vi "draw.vi"(0 "reference":refnum<class "PackageNode.lvclass">, 1 "graphics":refnum<class "Graphics.lvclass">, 5 "error in (no error)":errorcluster) -> (14 "reference out":refnum<class "PackageNode.lvclass">, 19 "error out":errorcluster)   [LabVIEW 2014, in "PackageNode.lvclass"]
doc: "public void draw(Graphics2D g2)"
uses:
  <resource>/Framework/Providers/Open_GDS/UML/PackageNode_class/PackageNode.lvclass
  <resource>/Framework/Providers/Open_GDS/UML/Graphics_class/Graphics.lvclass
  <resource>/Framework/Providers/Open_GDS/UML/General/Point/Point Point2D.ctl
  <resource>/Framework/Providers/Open_GDS/UML/MultiLineString_class/MultiLineString.lvclass
  <resource>/Framework/Providers/Open_GDS/UML/RectangularNode_class/RectangularNode.lvclass
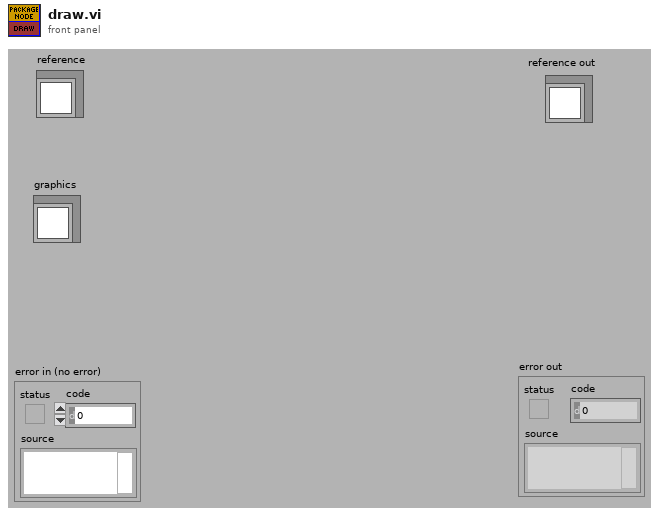
[diagram p1: front panel]
types:
  T1 = typedef "Point Point2D.ctl" = cluster{"x":dbl, "y":dbl}
  T2 = typedef "PackageNode.lvclass/ObjectAttributes.ctl" = cluster{"name":string, "contents":refnum<class "MultiLineString.lvclass">, "DEFAULT_TOP_WIDTH":i32, "DEFAULT_TOP_HEIGHT":i32, "DEFAULT_WIDTH":i32, "DEFAULT_HEIGHT":i32, "NAME_GAP":i32, "XGAP":i32, "YGAP":i32, "Collapsed":bool, "Note color":u32, "Justification":u16}
  T3 = typedef "RectangularNode.lvclass/ObjectAttributes.ctl" = cluster{"bounds":T4}
  T4 = typedef "Rectangle Rectangle2D.ctl" = cluster{"x":dbl, "y":dbl, "width":dbl, "height":dbl}
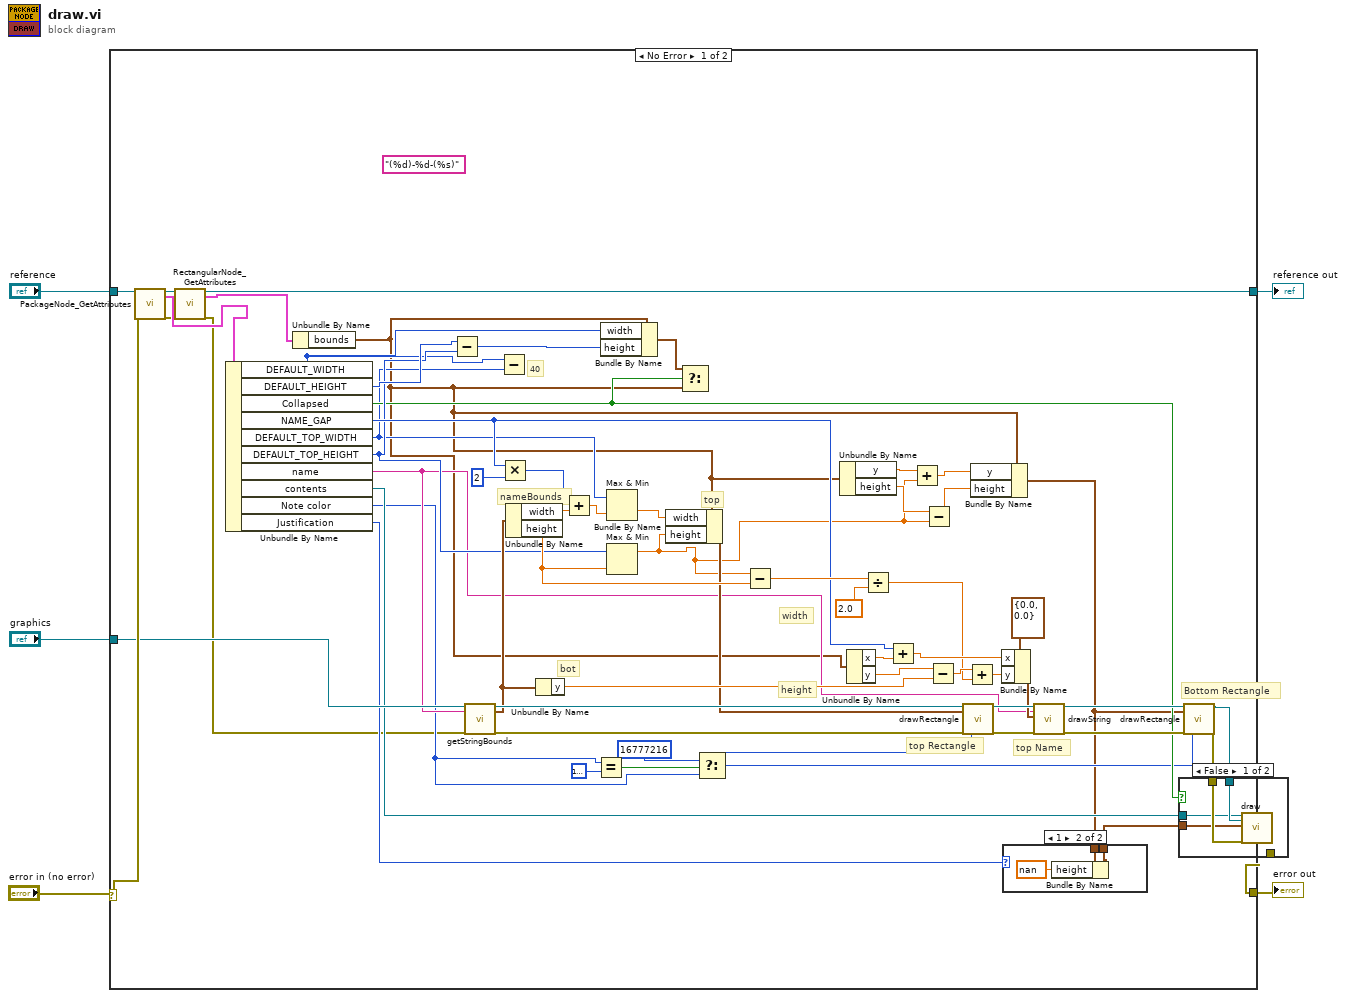
[diagram p0: block diagram]
diagram:
  n1 = case shown="No Error" "error in (no error)" {
    selector: "error in (no error)" -> [w64 w77]
    tunnel: "reference" -> [w66 w78]
    tunnel: [w65 w77] -> w4
    tunnel: [w7 w78] -> w3
    tunnel: "graphics" -> [w63 _]
    frame No Error {
      (unwired) "(%d)-%d-(%s)" ("format string")
      # "40"
      # "Bottom Rectangle"
      # "top Name"
      # "top Rectangle"
      # "height"
      # "width"
      # "bot"
      # "top"
      # "nameBounds"
      n2 = call <resource>:"PackageNode_GetAttributes.vi"("reference in"=w66, "error in (no error)"=w64) -> ("reference out"=w10:refnum<class "PackageNode.lvclass">, "Data"=w11:T2, "error out"=w9:errorcluster)  [unwired: 1 in, 14 out]
      n3 = call <resource>:"RectangularNode_GetAttributes.vi"("reference in"=w10, "error in (no error)"=w9) -> ("reference out"=w7:refnum<class "PackageNode.lvclass">, "Data"=w6:T3, "error out"=w8:errorcluster)  [unwired: 14 in, 1 out]
      n4 = Unbundle By Name(w11) -> ("DEFAULT_WIDTH"=w22:i32, "DEFAULT_HEIGHT"=w27:i32, "Collapsed"=w24:bool, "NAME_GAP"=w38:i32, "DEFAULT_TOP_WIDTH"=w21:i32, "DEFAULT_TOP_HEIGHT"=w26:i32, "name"=w23:string, "contents"=w29:refnum<class "MultiLineString.lvclass">, "Note color"=w16:u32, "Justification"=w12:u16)
      n5 = Unbundle By Name(w6) -> ("bounds"=w20:T4)
      n6 = Subtract(x=w27, y=w26) -> (x-y=w25:i32)
      n7 = call-dynamic "getStringBounds.vi"("reference"=w63, "text"=w23, "error in (no error)"=w8) -> ("reference out"=w60:refnum<class "Graphics.lvclass">, "bounds"=w36:T4, "error out"=w39:errorcluster)  [unwired: 14 in]
      n8 = Subtract(x=w22, y=w21) -> ()  [unwired: 1 out]
      n9 = Multiply(x=w38, y=2 ("x")) -> (x*y=w57:i32)
      n10 = Unbundle By Name(w36) -> ("width"=w58:dbl, "height"=w43:dbl)
      n11 = Unbundle By Name(w36) -> ("y"=w44:dbl)
      n12 = Add(x=w57, y=w58) -> (x+y=w56:dbl)
      n13 = Equal?(x=w16, y=u32 16777216) -> (x = y?=w18:bool)
      n14 = Bundle By Name(cluster=w20, "width"=w22, "height"=w25) -> (w28:T4)
      n15 = Max & Min(x=w21, y=w56) -> (max(x,y)=w59:dbl)  [unwired: 1 out]
      n16 = Max & Min(x=w26, y=w43) -> (max(x,y)=w31:dbl)  [unwired: 1 out]
      n17 = Bundle By Name(cluster=w20, "width"=w59, "height"=w31) -> (w35:T4)
      n18 = Select(t=w28, s=w24, f=w20) -> ()  [unwired: 1 out]
      n19 = Select(t=u32 16777216 ("FillClor(if not used=BorderColorIsUsed,AutoFill)"), s=w18, f=w16) -> (s? t:f=w15:u32)
      n20 = Subtract(x=w31, y=w43) -> (x-y=w42:dbl)
      n21 = Unbundle By Name(w20) -> ("y"=w34:dbl, "height"=w32:dbl)
      n22 = Unbundle By Name(w20) -> ("x"=w49:dbl, "y"=w45:dbl)
      n23 = Divide(x=w42, y=2.0) -> (x/y=w40:dbl)
      n24 = Add(x=w38, y=w49) -> (x+y=w48:dbl)
      n25 = Add(x=w34, y=w31) -> (x+y=w33:dbl)
      n26 = Subtract(x=w32, y=w31) -> (x-y=w30:dbl)
      n27 = Subtract(x=w45, y=w44) -> (x-y=w46:dbl)
      n28 = call <resource>:"drawRectangle.vi"("reference"=w60, "rectangle"=w35, "error in (no error)"=w39, "FillClor(if not used=BorderColorIsUsed,AutoFill)"=w15) -> ("reference out"=w55:refnum<class "Graphics.lvclass">, "error out"=w54:errorcluster)  [unwired: 3 in, 11 out]
      n29 = Add(x=w46, y=w40) -> (x+y=w47:dbl)
      n30 = Bundle By Name(cluster=w20, "y"=w33, "height"=w30) -> (w14:T4)
      n31 = Bundle By Name(cluster=T1 {"x"=0.0, "y"=0.0} ("textPos"), "x"=w48, "y"=w47) -> (w50:T1)
      n32 = case shown="1" w12 {
        tunnel: w14 -> [w67 w70]
        tunnel: [w67 w69] -> w13
        frame 0, Default {
        }
        frame 1 {
          n33 = Bundle By Name(cluster=w70, "height"=nan) -> (w69:T4)
        }
      }
      n34 = call-dynamic "drawString.vi"("reference"=w55, "text"=w23, "textPos"=w50, "error in (no error)"=w54) -> ("reference out"=w53:refnum<class "Graphics.lvclass">, "error out"=w52:errorcluster)  [unwired: 14 in]
      n35 = call <resource>:"drawRectangle.vi"("reference"=w53, "rectangle"=w14, "error in (no error)"=w52, "FillClor(if not used=BorderColorIsUsed,AutoFill)"=w15) -> ("reference out"=w62:refnum<class "Graphics.lvclass">, "error out"=w61:errorcluster)  [unwired: 3 in, 11 out]
      n36 = case shown="False" w24 {
        tunnel: [w75 w76] -> w65
        tunnel: w62 -> [w74 _]
        tunnel: w61 -> [w73 w76]
        tunnel: w13 -> [w72 _]
        tunnel: w29 -> [w71 _]
        frame False {
          n37 = call-dynamic "draw.vi"("reference"=w71, "graphics"=w74, "bounds"=w72, "error in (no error)"=w73) -> ("error out"=w75:errorcluster)  [unwired: 14 in, 1 out]
        }
        frame True {
        }
      }
    }
    frame Error {
    }
  }
  "reference out" <- w3
  "error out" <- w4
